vi "Persistent_XML_Read.vi"(8 "error in (no error)":errorcluster, 11 "Persistent XML File Path":path) -> (0 "error out":errorcluster, 3 "PersistentData":T1 {"RecircPumpFlow"."Recirc Pump Flow Set - R6" min=0.0 max=20.0; "RecircPumpFlow"."Recirc Pump Flow Set - R5" min=0.0 max=20.0; "RecircPumpFlow"."Recirc Pump Flow Set - R4" min=0.0 max=20.0; "RecircPumpFlow"."Recirc Pump Flow Set - R3" min=0.0 max=20.0; "RecircPumpFlow"."Recirc Pump Flow Set - R2" min=0.0 max=20.0; "RecircPumpFlow"."Recirc Pump Flow Set - R1" min=0.0 max=20.0; "MiniscusPressure"."Meniscus Pressure Set - R6" min=0.0 max=20.0; "MiniscusPressure"."Meniscus Pressure Set - R5" min=0.0 max=20.0; "MiniscusPressure"."Meniscus Pressure Set - R4" min=0.0 max=20.0; "MiniscusPressure"."Meniscus Pressure Set - R3" min=0.0 max=20.0; "MiniscusPressure"."Meniscus Pressure Set - R2" min=0.0 max=20.0; "MiniscusPressure"."Meniscus Pressure Set - R1" min=0.0 max=20.0; "Meniscus Vac Pump Speed" min=0.0 max=100.0})   [LabVIEW 2022 SP3]
uses:
  Controls/PersistentData--Cluster.ctl
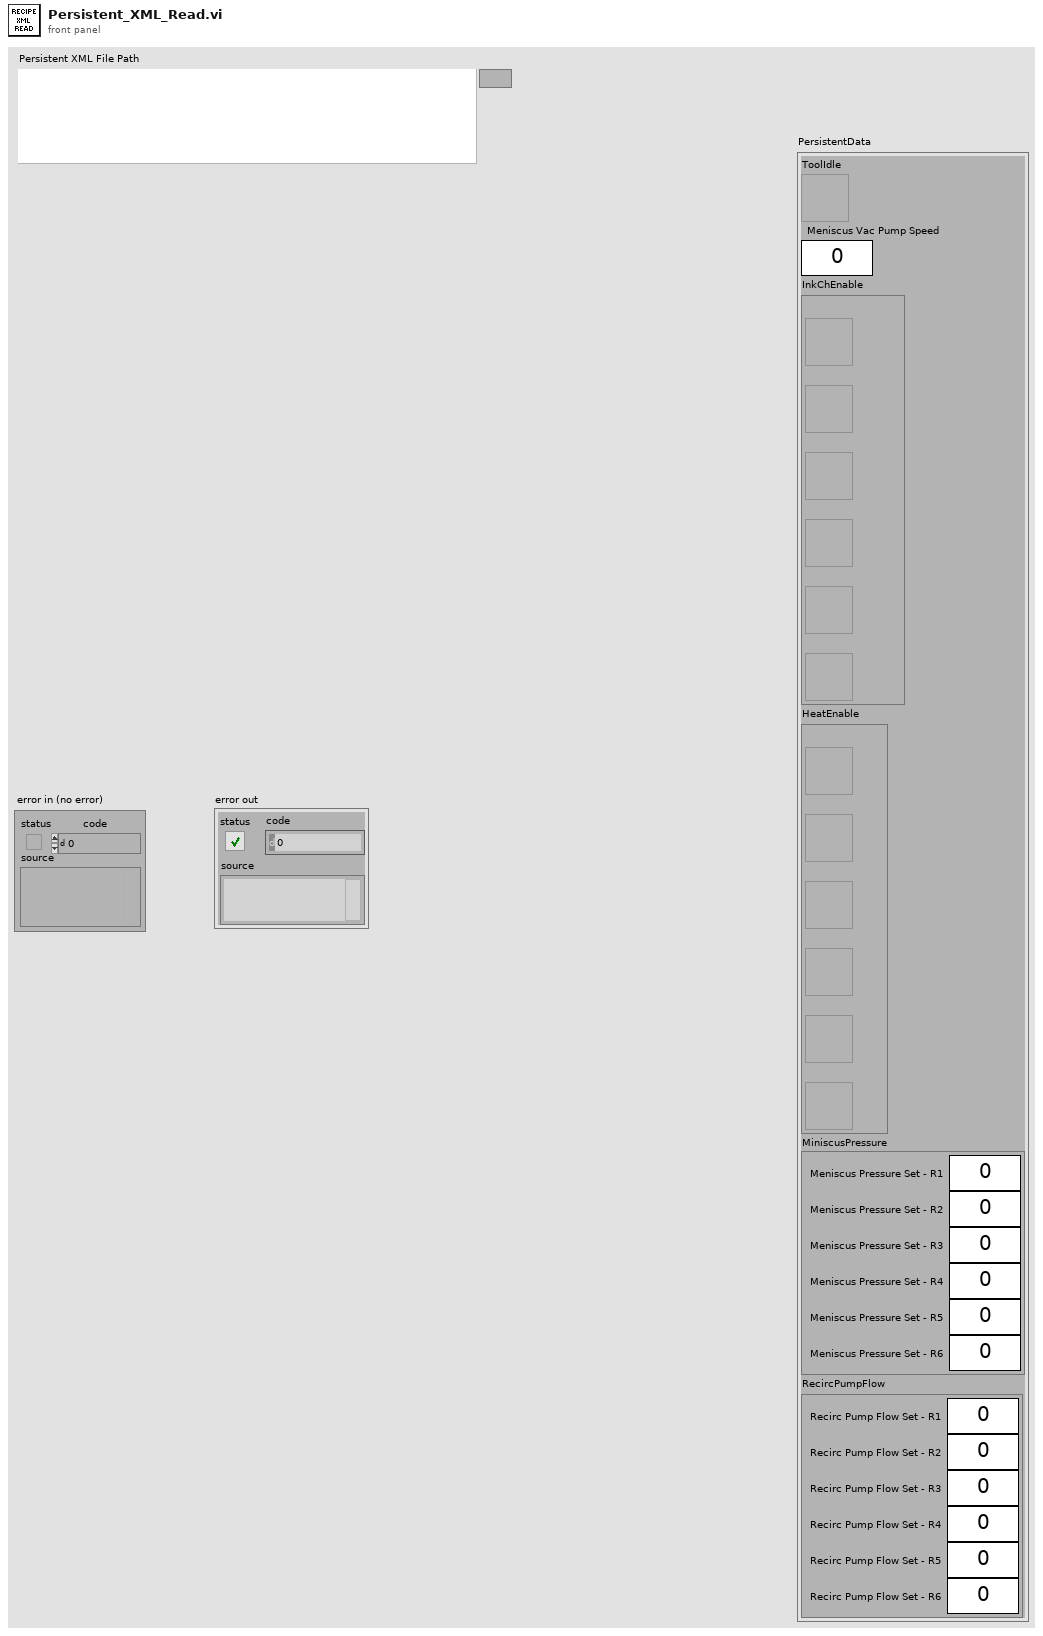
[diagram p1: front panel]
types:
  T1 = typedef "PersistentData--Cluster.ctl" = cluster{"ToolIdle":bool, "Meniscus Vac Pump Speed":dbl, "InkChEnable":cluster{"Enable Ink Ch-1":bool, "Enable Ink Ch-2":bool, "Enable Ink Ch-3":bool, "Enable Ink Ch-4":bool, "Enable Ink Ch-5":bool, "Enable Ink Ch-6":bool}, "HeatEnable":cluster{"Heater-1 Off":bool, "Heater-2 Off":bool, "Heater-3 Off":bool, "Heater-4 Off":bool, "Heater-5 Off":bool, "Heater-6 Off":bool}, "MiniscusPressure":cluster{"Meniscus Pressure Set - R1":dbl, "Meniscus Pressure Set - R2":dbl, "Meniscus Pressure Set - R3":dbl, "Meniscus Pressure Set - R4":dbl, "Meniscus Pressure Set - R5":dbl, "Meniscus Pressure Set - R6":dbl}, "RecircPumpFlow":cluster{"Recirc Pump Flow Set - R1":dbl, "Recirc Pump Flow Set - R2":dbl, "Recirc Pump Flow Set - R3":dbl, "Recirc Pump Flow Set - R4":dbl, "Recirc Pump Flow Set - R5":dbl, "Recirc Pump Flow Set - R6":dbl}}
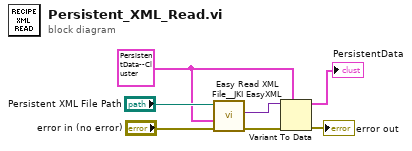
[diagram p0: block diagram]
diagram:
  w1 = T1 {"ToolIdle"=FALSE, "Meniscus Vac Pump Speed"=0.0, "InkChEnable"={"Enable Ink Ch-1"=FALSE, "Enable Ink Ch-2"=FALSE, "Enable Ink Ch-3"=FALSE, "Enable Ink Ch-4"=FALSE, "Enable Ink Ch-5"=FALSE, "Enable Ink Ch-6"=FALSE}, "HeatEnable"={"Heater-1 Off"=FALSE, "Heater-2 Off"=FALSE, "Heater-3 Off"=FALSE, "Heater-4 Off"=FALSE, "Heater-5 Off"=FALSE, "Heater-6 Off"=FALSE}, "MiniscusPressure"={"Meniscus Pressure Set - R1"=0.0, "Meniscus Pressure Set - R2"=0.0, "Meniscus Pressure Set - R3"=0.0, "Meniscus Pressure Set - R4"=0.0, "Meniscus Pressure Set - R5"=0.0, "Meniscus Pressure Set - R6"=0.0}, "RecircPumpFlow"={"Recirc Pump Flow Set - R1"=0.0, "Recirc Pump Flow Set - R2"=0.0, "Recirc Pump Flow Set - R3"=0.0, "Recirc Pump Flow Set - R4"=0.0, "Recirc Pump Flow Set - R5"=0.0, "Recirc Pump Flow Set - R6"=0.0}} ("PersistentData")
  n1 = call <vilib>:"Easy Read XML File__JKI EasyXML.vi"("error in (no error)"="error in (no error)", "LabVIEW Data (Type)"=w1, "XML File Path"="Persistent XML File Path") -> ("error out"=w4:errorcluster, "LabVIEW Data"=w5:variant)  [unwired: 6 in, 1 out]
  n2 = Variant To Data(error in=w4, type=w1, Variant=w5) -> (data=→"PersistentData":T1, error out=→"error out":errorcluster)
